vi "Max and Min.vi"   [LabVIEW 2019, in "xy_utilities.lvlib"]
doc: "Returns (x,y) coordinates of <b>y_max</b> and <b>y_min</b>.\n\nWire data to the data input to determine the polymorphic instance to use or manually select the instance."
uses:
  xy_utilities.lvlib
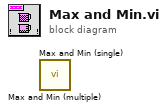
[diagram p0: block diagram]
diagram:
  n1 = call "Max and Min (multiple).vi"() -> ()  [unwired: 8 in, 4 out]
  n2 = call "Max and Min (single).vi"() -> ()  [unwired: 8 in, 4 out]
